vi "Remove Residue from Denominator.vi"   [LabVIEW 2017, in "NI_AALPro.lvlib"]
doc: "Removes the residue from the denominator if the numerator equals zero. The data types you wire to the <B>Numerator</B> and <B>Denominator</B> inputs determine the polymorphic instance to use."
uses:
  <vilib>/Analysis/NI_AALPro.lvlib
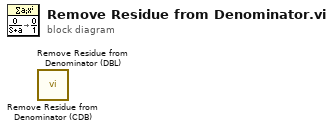
[diagram p0: block diagram]
diagram:
  n1 = call <vilib>:"Remove Residue from Denominator (CDB).vi"() -> ()  [unwired: 9 in, 3 out]
  n2 = call <vilib>:"Remove Residue from Denominator (DBL).vi"() -> ()  [unwired: 9 in, 3 out]
